vi "plotter save png.vi"(6 "binned plotter png save path":path, 9 "plotter png save path":path, 10 "XYGraph Refnum in":refnum<vi>, 11 "XYGraph in":refnum<vi>) -> ()   [LabVIEW 2013]
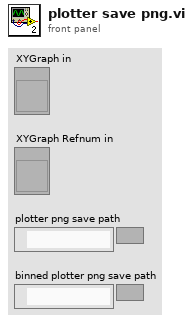
[diagram p1: front panel]
types:
  T1 = typedef "imagedata.ctl" = cluster{"image type":i32, "image depth":i32, "image":u8[], "mask":u8[], "colors":u32[], "Rectangle":cluster{"left":i16, "top":i16, "right":i16, "bottom":i16}}
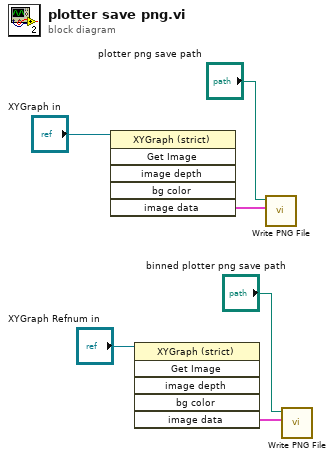
[diagram p0: block diagram]
diagram:
  n1 = invoke on="Invoke Node" class="XYGraph (strict)" method="Get Image"(reference="XYGraph in") -> ("image data"=w3:T1)  [unwired: 5 in, 5 out]
  n2 = invoke on="Invoke Node" class="XYGraph (strict)" method="Get Image"(reference="XYGraph Refnum in") -> ("image data"=w4:T1)  [unwired: 5 in, 5 out]
  n3 = call <vilib>:"Write PNG File.vi"("image data"=w3, "path to PNG file"="plotter png save path") -> ()  [unwired: 8 in, 2 out]
  n4 = call <vilib>:"Write PNG File.vi"("image data"=w4, "path to PNG file"="binned plotter png save path") -> ()  [unwired: 8 in, 2 out]
